vi "Find some Public API VI.vi"(7 "App Ref":refnum<vi>, 8 "Public Api file index":i32, 10 "Theme":bool=TRUE, 11 "Library in":refnum<vi>) -> ()   [LabVIEW 2019, in "Panther Dashboard.lvlib"]
uses:
  Panther Dashboard.lvlib
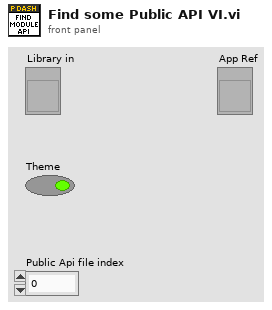
[diagram p1: front panel]
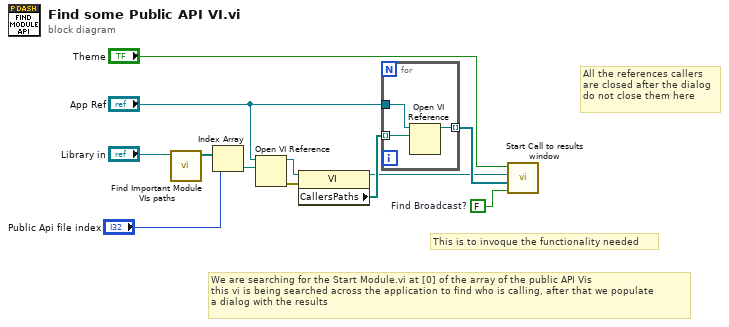
[diagram p0: block diagram]
diagram:
  w2 = FALSE  # Find Broadcast?
  # "All the references callers\nare closed after the dialog\ndo not close them here"
  # "This is to invoque the functionality needed"
  # "We are searching for the Start Module.vi at [0] of the array of the public API Vis\nthis vi is being searched across the application to find who is calling, after that we populate\na dialog with the results"
  n1 = call "Find Important Module VIs paths.vi"("Library in"="Library in") -> ("Public API VIs Paths"=w10:path[])  [unwired: 10 in]
  n2 = Index Array(array=w10, index="Public Api file index") -> (element=w9:path)
  n3 = Open VI Reference(application reference (local)="App Ref", vi path=w9) -> (vi reference=w8:refnum<vi>, error out=w12:errorcluster)  [unwired: 4 in]
  n4 = property class="VI"(reference=w8, error in=w12) -> (reference out=w4:refnum<vi>, "CallersPaths"=w6:path[])  [unwired: 1 out]
  n5 = for {
    tunnel: "App Ref" -> [w15]
    tunnel: w6 -> [w14] mode=indexing
    tunnel: [w13] -> w5 mode=indexing
    n6 = Open VI Reference(application reference (local)=w15, vi path=w14) -> (vi reference=w13:refnum<vi>)  [unwired: 4 in, 1 out]
  }
  n7 = call "Start Call to results window.vi"("Find Broadcast?"=w2, "Request VI Callers"=w5, "Event"=w4, "Theme"="Theme") -> ()  [unwired: 8 in]
